vi "Log.vi"(8 "error in":errorcluster, 11 "SDO Transfer in":refnum<class "SDO Transfer.lvclass">) -> (0 "error out":errorcluster, 3 "SDO Transfer out":refnum<class "SDO Transfer.lvclass">)   [LabVIEW 2020, in "CANopen.lvlib" / "SDO Manager.lvlib" / "SDO Transfer.lvclass"]
uses:
  SDO Transfer.lvclass
  SDO Transfer.lvclass/SDO Transfer.ctl
  Logging/Log Level.vi
  Logging/CANopen Logging.lvlib
  <resource>/AFDebug/AF Debug.lvlib
  <vilib>/Utility/SystemLogging/NI_SystemLogging.lvlib
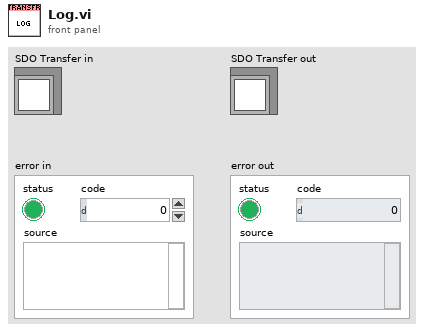
[diagram p1: front panel]
types:
  T1 = enum16{"Error", "Warn", "Info", "Debug", "Trace"}
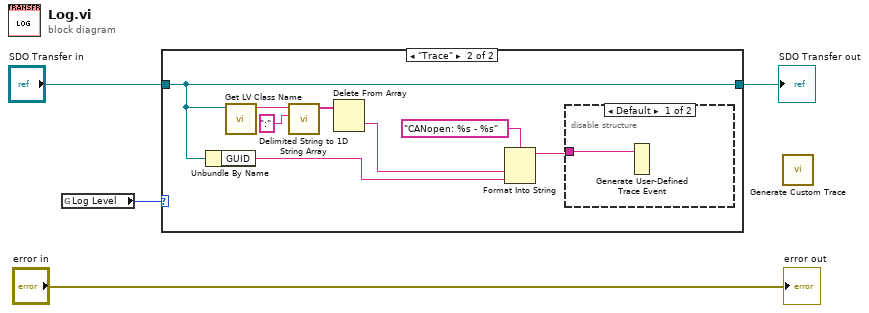
[diagram p0: block diagram]
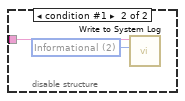
[diagram p3: hidden frame]
diagram:
  n1 = global read "Log Level.vi" "Log Level"() -> (w3:T1)
  n2 = case shown="\"Trace\"" w3 {
    tunnel: "SDO Transfer in" -> [w5 w10]
    tunnel: [w5 w10] -> w4
    frame Default {
    }
    frame "Trace" {
      n3 = Unbundle By Name(w10) -> ("GUID"=w8:string)
      n4 = call <vilib>:"Get LV Class Name.vi"("object"=w10) -> ("class name"=w13:string)  [unwired: 9 in, 1 out]
      n5 = call <vilib>:"Delimited String to 1D String Array.vi"("delimiter"=":", "delimited string"=w13) -> ("string array"=w12:string[])  [unwired: 9 in]
      n6 = Delete From Array(array=w12) -> (deleted portion=w9:string)  [unwired: 2 in, 1 out]
      n7 = Format Into String(format string="CANopen: %s - %s", w9, w8) -> (resulting string=w6:string)  [unwired: 2 in, 1 out]
      n8 = disable-structure shown="Default" {
        disable-tunnel: w6 -> [w14 w16]
        frame condition #0 (active) {
          n9 = Generate User-Defined Trace Event(2:w14) -> ()  [unwired: 1 in]
        }
        frame condition #1 {
          w15 = 2 items=["Error", "Warning", "Informational"] ("severity")
          n10 = call <vilib>:"Write to System Log.vi"("severity"=w15, "message"=w16) -> ()  [unwired: 9 in, 1 out]
        }
      }
    }
  }
  "SDO Transfer out" <- w4
  n11 = call <resource>:"Generate Custom Trace.vi"() -> ()  [unwired: 12 in]
  "error out" <- "error in"
